vi "Erase Rx Message.vi"(8 "error in (no error)":errorcluster, 11 "AutoExp in":refnum<class "AutoExp.lvclass">) -> (0 "error out":errorcluster, 3 "AutoExp out":refnum<class "AutoExp.lvclass">)   [LabVIEW 2018, in "AutoExp.lvclass"]
uses:
  AutoExp.lvclass
  AutoExp.lvclass/AutoExp.ctl
  Channel/Channel.lvclass
  RxTx/RxTx.lvclass
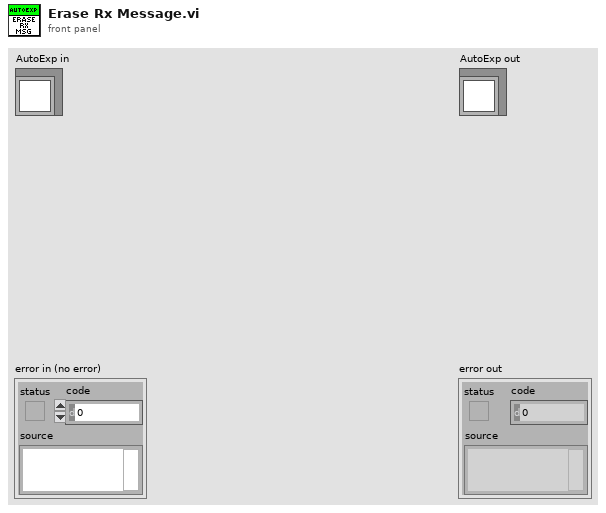
[diagram p1: front panel]
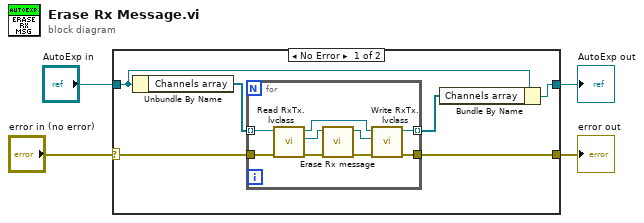
[diagram p0: block diagram]
diagram:
  n1 = case shown="No Error" "error in (no error)" {
    selector: "error in (no error)" -> [w8 w21]
    tunnel: [w7 w21] -> w3
    tunnel: [w9 w20] -> w1
    tunnel: "AutoExp in" -> [w10 w20]
    frame No Error {
      n2 = Unbundle By Name(w10) -> ("Channels array"=w6:refnum<class "Channel.lvclass">[])
      n3 = for {
        tunnel: w8 -> [w19]
        tunnel: [w18] -> w7
        tunnel: w6 -> [w17] mode=indexing
        tunnel: [w16] -> w5 mode=indexing
        n4 = call "Read RxTx.lvclass.vi"("error in (no error)"=w19, "Channel in"=w17) -> ("error out"=w12:errorcluster, "RxTx.lvclass"=w15:refnum<class "RxTx.lvclass">, "Channel out"=w11:refnum<class "Channel.lvclass">)  [unwired: 7 in]
        n5 = call "Erase Rx message.vi"("error in (no error)"=w12, "RxTx in"=w15) -> ("error out"=w13:errorcluster, "RxTx out"=w14:refnum<class "RxTx.lvclass">)  [unwired: 8 in]
        n6 = call "Write RxTx.lvclass.vi"("error in (no error)"=w13, "RxTx.lvclass"=w14, "Channel in"=w11) -> ("error out"=w18:errorcluster, "Channel out"=w16:refnum<class "Channel.lvclass">)  [unwired: 7 in]
      }
      n7 = Bundle By Name(cluster=w10, "Channels array"=w5) -> (w9:refnum<class "AutoExp.lvclass">)
    }
    frame Error {
    }
  }
  "error out" <- w3
  "AutoExp out" <- w1
